vi "Pixel Clock Control.vi"(10 "Pixel time (tick)":i32, 11 "Pixel clock_pulse width":i32) -> (2 "Pixel time":i32, 3 "Pixel time up":bool)   [LabVIEW 2015]
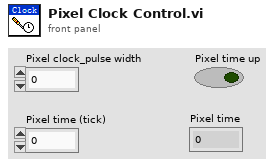
[diagram p1: front panel]
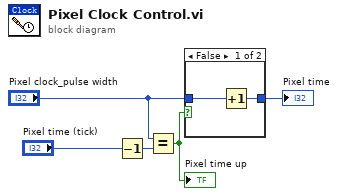
[diagram p0: block diagram]
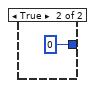
[diagram p2: hidden frame]
diagram:
  n1 = Decrement(x="Pixel time (tick)") -> (x-1=w3:i32)
  n2 = Equal?(x="Pixel clock_pulse width", y=w3) -> (x = y?=w4:bool)
  "Pixel time up" <- w4
  n3 = case shown="False" w4 {
    tunnel: "Pixel clock_pulse width" -> [w7 _]
    tunnel: [w6 0] -> w5
    frame False {
      n4 = Increment(x=w7) -> (x+1=w6:i32)
    }
    frame True {
    }
  }
  "Pixel time" <- w5
